vi "Calc_PEarson_Coeff.vi"(10 "Y":sgl[](array[numeric]), 11 "X":sgl[](array[numeric])) -> (3 "R":sgl)   [LabVIEW 2020]
uses:
  <vilib>/Analysis/baseanly.llb/Mean (DBL).vi
  <vilib>/Analysis/NI_AALBase.lvlib
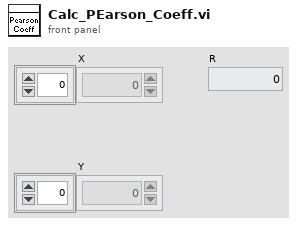
[diagram p1: front panel]
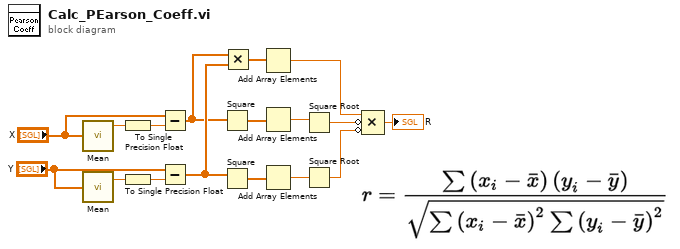
[diagram p0: block diagram]
diagram:
  n1 = call-poly <vilib>:"Mean.vi"("X"="X") -> ("mean"=w2:dbl)  [unwired: 1 out]
  n2 = call-poly <vilib>:"Mean.vi"("X"="Y") -> ("mean"=w4:dbl)  [unwired: 1 out]
  n3 = To Single Precision Float(number=w2) -> (single precision float=w3:sgl)
  n4 = To Single Precision Float(number=w4) -> (single precision float=w5:sgl)
  n5 = Subtract(x="X", y=w3) -> (x-y=w7:sgl[])
  n6 = Subtract(x="Y", y=w5) -> (x-y=w8:sgl[])
  n7 = Square(x=w7) -> (x^2=w9:sgl[])
  n8 = Square(x=w8) -> (x^2=w10:sgl[])
  n9 = Multiply(x=w7, y=w8) -> (x*y=w11:sgl[])
  n10 = Add Array Elements(numeric array=w11) -> (sum=w14:sgl)
  n11 = Add Array Elements(numeric array=w9) -> (sum=w12:sgl)
  n12 = Add Array Elements(numeric array=w10) -> (sum=w13:sgl)
  n13 = Square Root(x=w12) -> (sqrt(x)=w15:sgl)
  n14 = Square Root(x=w13) -> (sqrt(x)=w16:sgl)
  n15 = Compound Arithmetic op=MULTIPLY(w14, invert w15, invert w16) -> (→"R":sgl)
